vi "Configure Power Factor Limits.vi"(0 "VISA resource name":refnum<visa-resource-name>, 5 "Power Factor Low Limit (0)":dbl min=0.0 max=1.0 format="%.3f", 7 "Power Factor High Limit (0)":dbl min=0.0 max=1.0 format="%.3f", 11 "error in (no error)":errorcluster) -> (4 "VISA resource name out":refnum<visa-resource-name>, 15 "error out":errorcluster)   [LabVIEW 2020, in "eec 6700.lvlib"]
doc: "Configures the power factor limits in the active step of the power source instrument.\n\nPower Factor Limit setting configures a minimum and maximum threshold level. If a minimum level is not reached a test failure will occur. If a maximum level is reached a test failure will occur."
uses:
  <instrlib>/eec 6700/eec 6700.lvlib
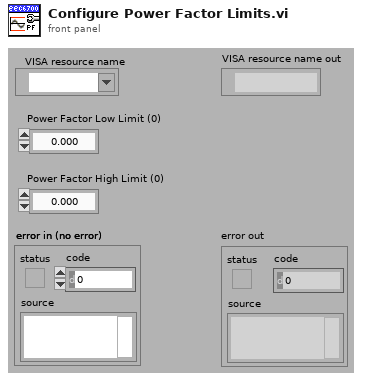
[diagram p1: front panel]
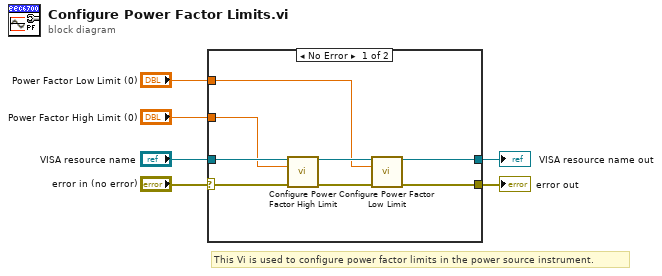
[diagram p0: block diagram]
diagram:
  # "This Vi is used to configure power factor limits in the power source instrument."
  n1 = case shown="No Error" "error in (no error)" {
    selector: "error in (no error)" -> [w9 w16]
    tunnel: [w13 w16] -> w6
    tunnel: [w12 w15] -> w5
    tunnel: "VISA resource name" -> [w10 w15]
    tunnel: "Power Factor High Limit (0)" -> [w8 _]
    tunnel: "Power Factor Low Limit (0)" -> [w7 _]
    frame No Error {
      n2 = call <instrlib>:"Configure Power Factor High Limit.vi"("VISA resource name"=w10, "Power Factor High Limit (0)"=w8, "error in (no error)"=w9) -> ("VISA resource name out"=w11:refnum<visa-resource-name>, "error out"=w14:errorcluster)  [unwired: 11 in]
      n3 = call <instrlib>:"Configure Power Factor Low Limit.vi"("VISA resource name"=w11, "Power Factor Low Limit (0)"=w7, "error in (no error)"=w14) -> ("VISA resource name out"=w12:refnum<visa-resource-name>, "error out"=w13:errorcluster)  [unwired: 11 in]
    }
    frame Error {
    }
  }
  "error out" <- w6
  "VISA resource name out" <- w5
